vi "MFC_Data_Process.vi"(0 "MFC":dbl[](array[numeric])) -> (4 "MFC Absolute Pressure":string, 6 "MFC Temperature":string, 8 "MFC Volumetric Flow":string, 10 "MFC Mass Flow":string, 15 "MFC Set Point":string)   [LabVIEW 2014]
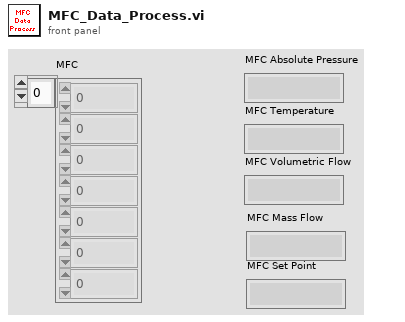
[diagram p1: front panel]
types:
  T1 = cluster{"[0]":string, "[1]":string, "[2]":string, "[3]":string, "[4]":string, "[5]":string, "[6]":string, "[7]":string, "[8]":string}
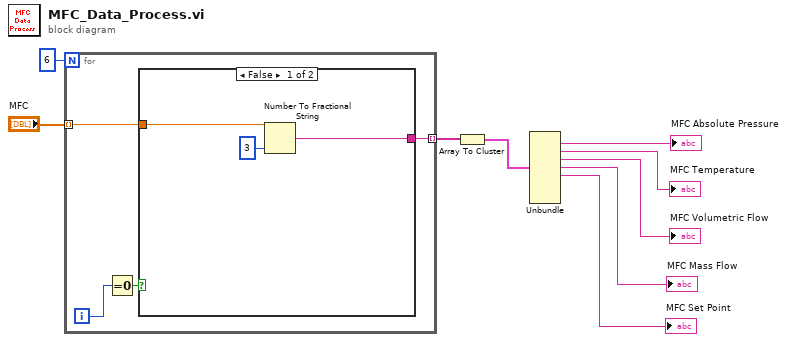
[diagram p0: block diagram]
diagram:
  n1 = for {
    N: 6 -> [_]
    tunnel: "MFC" -> [w11] mode=indexing
    tunnel: [w10] -> w7 mode=indexing
    i -> [w13]
    n2 = Equal To 0?(x=w13) -> (x = 0?=w12:bool)
    n3 = case shown="False" w12 {
      tunnel: w11 -> [w15 _]
      tunnel: [w14 _] -> w10
      frame False {
        n4 = Number To Fractional String(number=w15, precision (6)=i16 3) -> (F-format string=w14:string)  [unwired: 2 in]
      }
      frame True {
        # "Skip the first element in array"
      }
    }
  }
  n5 = Array To Cluster(array=w7) -> (cluster=w6:T1)
  n6 = Unbundle(w6) -> ("[1]"=→"MFC Absolute Pressure":string, "[2]"=→"MFC Temperature":string, "[3]"=→"MFC Volumetric Flow":string, "[4]"=→"MFC Mass Flow":string, "[5]"=→"MFC Set Point":string)  [unwired: 4 out]
